vi "Initialize.vi"(8 "error in (no error)":errorcluster, 10 "Temp Conotroller Config":T1={"COM Port"="COM14", "Type"=enum."Disabled"}, 11 "TC-720 in":refnum<class "TC-720.lvclass">) -> (0 "error out":errorcluster, 3 "TC-720 out":refnum<class "TC-720.lvclass">)   [LabVIEW 2023, in "TC-720.lvlib" / "TC-720.lvclass"]
uses:
  TC-720.lvclass
  Resources/Type Defs/Temp Controller Configuration.ctl
  Temperature Controller/Temperature Controller.lvclass
  TC-720.lvclass/TC-720.ctl
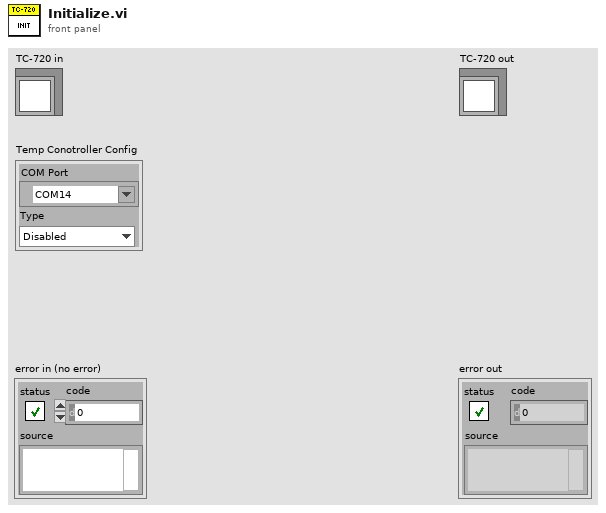
[diagram p1: front panel]
types:
  T1 = typedef "Temp Controller Configuration.ctl" = cluster{"COM Port":refnum<visa-resource-name>, "Type":enum16{"Disabled", "TC-720"}}
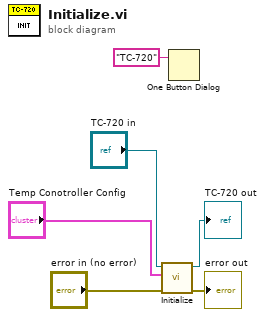
[diagram p0: block diagram]
diagram:
  n1 = call-parent "Initialize.vi"("error in (no error)"="error in (no error)", "Temp Conotroller Config"="Temp Conotroller Config", "Temperature Controller in"="TC-720 in") -> ("error out"=→"error out":errorcluster, "Temperature Controller out"=→"TC-720 out":refnum<class "TC-720.lvclass">)  [unwired: 7 in]
  n2 = One Button Dialog(message="TC-720") -> ()  [unwired: 1 in, 1 out]
